vi "Init Server.vi"(5 "EventLogger":refnum<class "EventLoggingService.lvclass">, 7 "SequenceCountService":refnum<class "SequenceCountService.lvclass">, 8 "error in (no error)":errorcluster, 9 "Bind Port":u16, 10 "IP Resolver":refnum<class "IP Resolver.lvclass">, 11 "Server Info":T1) -> (0 "error out":errorcluster, 3 "TCPMessaging out":refnum<class "TCPMessaging.lvclass">)   [LabVIEW 2020, in "Vecto.lvlib" / "TCPMessaging.lvclass"]
uses:
  TCPMessaging.lvclass
  SequenceCountService/SequenceCountService.lvclass
  EventLoggingService/EventLoggingService.lvclass
  proto/TcpClientInfo/Data.ctl
  TCP Mode.ctl
  Event Level.ctl
  TCPMessaging.lvclass/TCPMessaging.ctl
  EventLoggingService/EventLoggingService.lvclass/EventLoggingService.ctl
  <vilib>/Utility/error.llb/Error Cluster From Error Code.vi
  EventLogHandler/EventLogHandler.lvclass
  Vecto.lvlib
  proto/TcpClientInfo/TcpClientInfo.lvlib
  IP Resolver/IP Resolver.lvclass
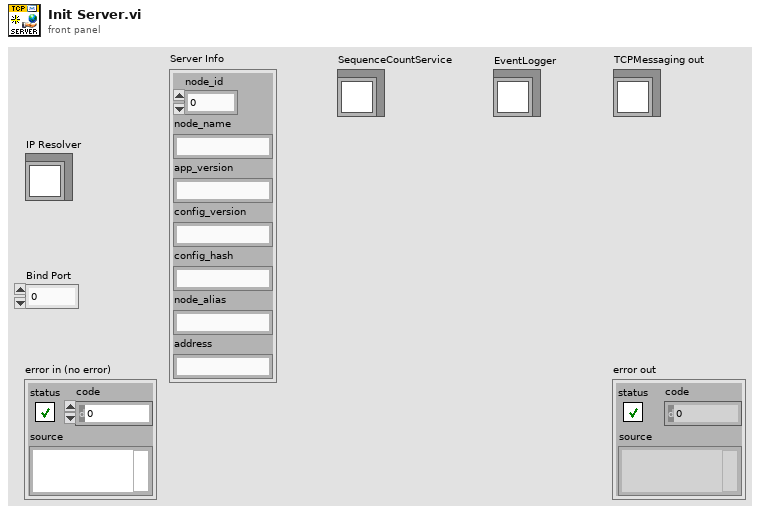
[diagram p1: front panel]
types:
  T1 = typedef "TcpClientInfo.lvlib/Data.ctl" = cluster{"node_id":u32, "node_name":string, "app_version":string, "config_version":string, "config_hash":string, "node_alias":string, "address":string}
  T2 = typedef "Vecto.lvlib/Event Level.ctl" = enum16{"Debug", "Info", "Warning", "Error"}
  T3 = typedef "Vecto.lvlib/TCPMessaging.lvclass/TCP Mode.ctl" = enum16{"Client", "Server"}
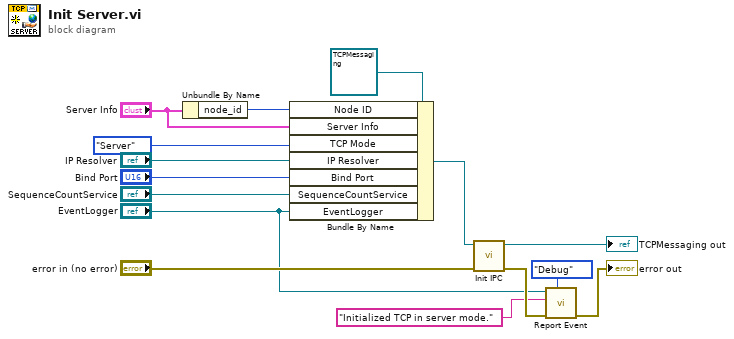
[diagram p0: block diagram]
diagram:
  n1 = Unbundle By Name("Server Info") -> ("node_id"=w3:u32)
  n2 = Bundle By Name(cluster=refnum<class "TCPMessaging.lvclass"> refnum ("TCPMessaging in"), "Node ID"=w3, "Server Info"="Server Info", "TCP Mode"=TCP_Mode."Server", "IP Resolver"="IP Resolver", "Bind Port"="Bind Port", "SequenceCountService"="SequenceCountService", "EventLogger"="EventLogger") -> (w11:refnum<class "TCPMessaging.lvclass">)
  n3 = call "Init IPC.vi"("error in (no error)"="error in (no error)", "TCPMessaging in"=w11) -> ("error out"=w12:errorcluster, "TCPMessaging out"=→"TCPMessaging out":refnum<class "TCPMessaging.lvclass">)  [unwired: 8 in]
  n4 = call "Report Event.vi"("Event Level (Info)"=Event_Level."Debug", "error in (no error)"=w12, "Message"="Initialized TCP in server mode.", "EventLoggingService in"="EventLogger") -> ("error out"=→"error out":errorcluster)  [unwired: 6 in, 1 out]
